vi "Update ROI times.vi"(11 "ROI setup in":T1[](array[typedef]) {"Apparent Frame Size" format="%#_6f"; "Original FOV (um)" format="%#_6f"; "Pixels per miniscan" format="%#_6f"; "Dwell Time per pixel" format="%#_6f"; "Resolution" format="%#_6f"; "ROI group ID" format="%#_6f"; "Laser Power (%)" format="%#_6f"; "Zoom" format="%#_6f"; "Frame Size" format="%#_6f"; "Number of lines" format="%#_6f"; "Composite ID" format="%#_6f"; "Angle (deg)" format="%#_6f"; "ROI Time (ns)" format="%#_6f"; "ROI ID" format="%#_6f"; "Pixels in ROI" format="%#_6f"; "ROI index" format="%#_6f"; "Z stop" format="%#_6f"; "Y stop" format="%#_6f"; "X stop" format="%#_6f"; "Z start" format="%#_6f"; "X start" format="%#_6f"; "Y start" format="%#_6f"}) -> (3 "ROI setup out":T1[](array[typedef]) {"Apparent Frame Size" format="%#_6f"; "Original FOV (um)" format="%#_6f"; "Pixels per miniscan" format="%#_6f"; "Dwell Time per pixel" format="%#_6f"; "Resolution" format="%#_6f"; "ROI group ID" format="%#_6f"; "Laser Power (%)" format="%#_6f"; "Zoom" format="%#_6f"; "Frame Size" format="%#_6f"; "Number of lines" format="%#_6f"; "Composite ID" format="%#_6f"; "Angle (deg)" format="%#_6f"; "ROI Time (ns)" format="%#_6f"; "ROI ID" format="%#_6f"; "Pixels in ROI" format="%#_6f"; "ROI index" format="%#_6f"; "Z stop" format="%#_6f"; "Y stop" format="%#_6f"; "X stop" format="%#_6f"; "Z start" format="%#_6f"; "X start" format="%#_6f"; "Y start" format="%#_6f"})   [LabVIEW 2020]
uses:
  Visualisation/Functional Imaging Viewer/Typedefs/ROI parameters data type.ctl
  Typedefs/ROI ID Enum.ctl
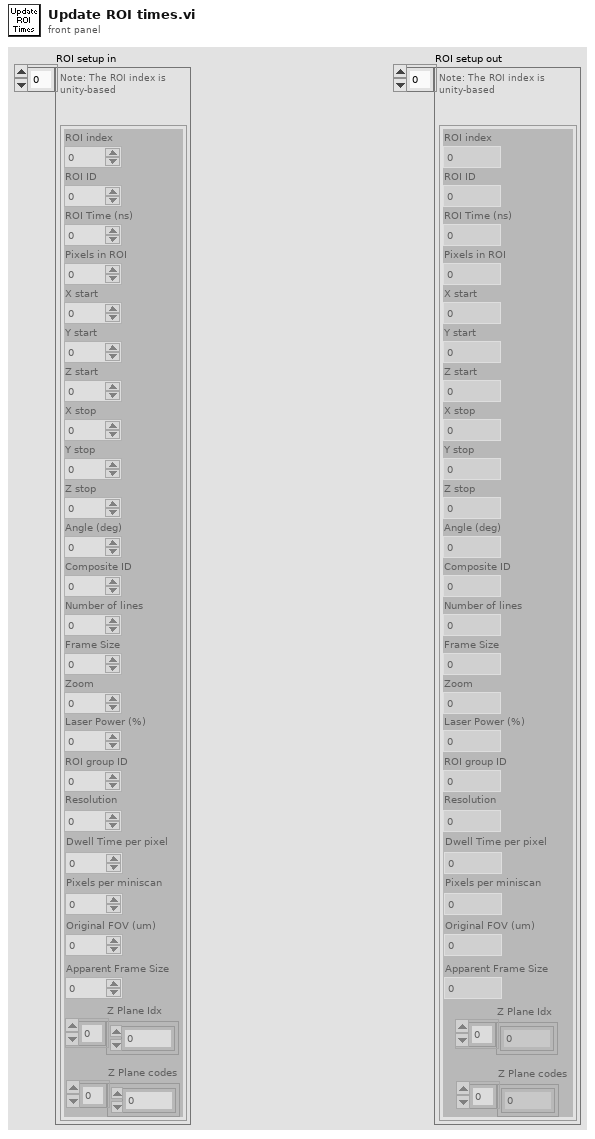
[diagram p1: front panel]
types:
  T1 = typedef "ROI parameters data type.ctl" = cluster{"ROI index":dbl, "ROI ID":dbl, "ROI Time (ns)":dbl, "Pixels in ROI":dbl, "X start":dbl, "Y start":dbl, "Z start":dbl, "X stop":dbl, "Y stop":dbl, "Z stop":dbl, "Angle (deg)":dbl, "Composite ID":dbl, "Number of lines":dbl, "Frame Size":dbl, "Zoom":dbl, "Laser Power (%)":dbl, "ROI group ID":dbl, "Resolution":dbl, "Dwell Time per pixel":dbl, "Pixels per miniscan":dbl, "Original FOV (um)":dbl, "Apparent Frame Size":dbl, "Z Plane Idx":i32[], "Z Plane codes":i32[]}
  T2 = typedef "ROI ID Enum.ctl" = enum16{"Point", "MiniScan", "Comp. MiniScan", "Rectangle", "Comp. volume", "Arb. plane point", "None"}
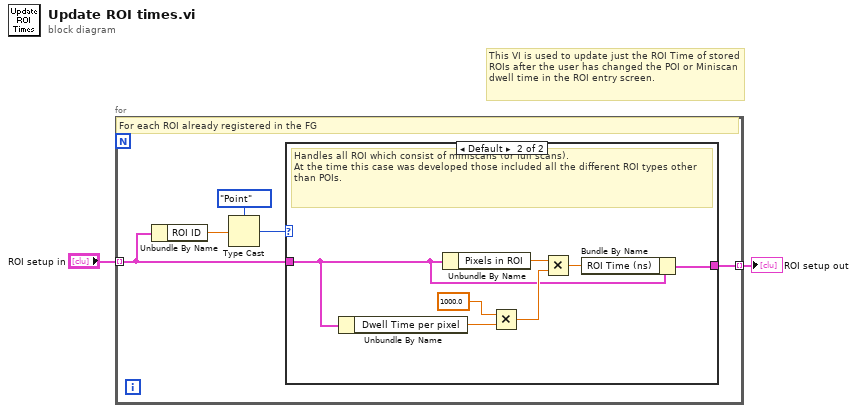
[diagram p0: block diagram]
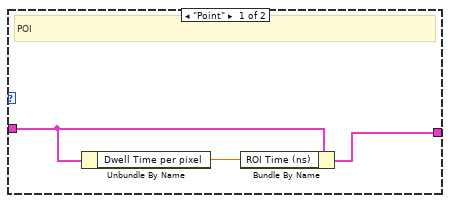
[diagram p2: hidden frame]
diagram:
  # "This VI is used to update just the ROI Time of stored ROIs after the user has changed the POI or Miniscan dwell time in the ROI entry screen."
  n1 = for {
    tunnel: "ROI setup in" -> [w3] mode=indexing
    tunnel: [w7] -> w1 mode=indexing
    # "For each ROI already registered in the FG"
    n2 = Unbundle By Name(w3) -> ("ROI ID"=w5:dbl)
    n3 = Type Cast(type=ROI_ID_Enum."Point" ("ROI Type"), x=w5) -> (*(type *) &x=w4:T2)
    n4 = case shown="Default" w4 {
      tunnel: [w10 w16] -> w7
      tunnel: w3 -> [w9 w12]
      frame "Point" {
        # "POI"
        n5 = Unbundle By Name(w9) -> ("Dwell Time per pixel"=w8:dbl)
        n6 = Bundle By Name(cluster=w9, "ROI Time (ns)"=w8) -> (w10:T1)
      }
      frame Default {
        # "Handles all ROI which consist of miniscans (or full scans).\nAt the time this case was developed those included all the different ROI types other than POIs."
        n7 = Unbundle By Name(w12) -> ("Dwell Time per pixel"=w11:dbl)
        n8 = Unbundle By Name(w12) -> ("Pixels in ROI"=w14:dbl)
        n9 = Multiply(x=1000.0, y=w11) -> (x*y=w13:dbl)
        n10 = Multiply(x=w14, y=w13) -> (x*y=w17:dbl)
        n11 = Bundle By Name(cluster=w12, "ROI Time (ns)"=w17) -> (w16:T1)
      }
    }
  }
  "ROI setup out" <- w1
